vi "WriteString.vi"(8 "Uart Input":cluster{u64} {"?" format="%x"}, 10 "String Data":string="LabVIEW Serial Port v3.0\r\nAsst.Prof.Dr.Santi Nuratch\r\nEmbedded Computing and Control Laboratory.\r\nECC-Lab@INC-KMUTT.\r\n" caption="Staring Data", 11 "Error Input":errorcluster) -> (0 "Uart Output":cluster{u64} {"?" format="%x"}, 2 "Bytes Written":u32, 3 "Error Output":errorcluster)   [LabVIEW 2019]
doc: "<B>Write</B> the <B>String Data</B> to the serial port."
uses:
  dll/LabViewUart.dll
panel:
  # "Write a string data to the serial port"
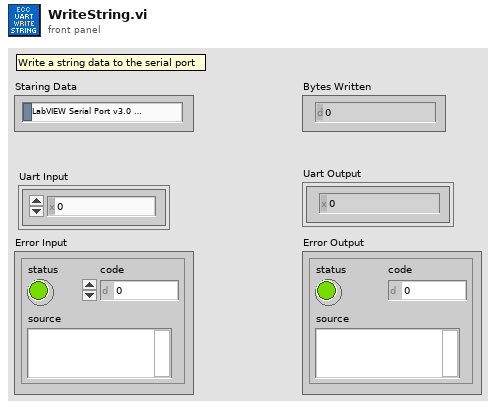
[diagram p1: front panel]
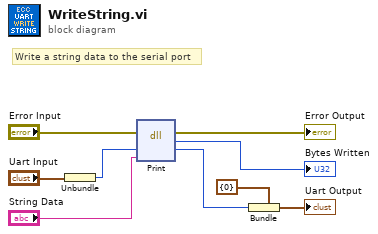
[diagram p0: block diagram]
diagram:
  # "Write a string data to the serial port"
  n1 = Unbundle("Uart Input") -> (w3:u64)
  n2 = dll-call lib="C:/uart-cmdex/SubVI/dll/LabViewUart.dll" fn="Print"(error in="Error Input", "Object Handle"=w3, "Data"="String Data") -> (error out=→"Error Output":errorcluster, "Bytes Written"=→"Bytes Written":u32, "Object Handle"=w2:u64)  [unwired: 3 in, 1 out]
  n3 = Bundle(cluster=cluster{u64} {0}, w2) -> (→"Uart Output":cluster{u64})
